vi "PrechargeCurrent.vi"(0 "Storage Voltage In (SP)":sgl format="%#_13g", 1 "Reinitialize":bool=TRUE, 2 "GainP":dbl=0.008 format="%#_13g", 3 "GainI":dbl=0.1 format="%#_13g", 5 "Drive Voltage In (PV)":sgl format="%#_13g", 7 "Setpoint High":dbl=100.0, 9 "Setpoint Low":dbl, 11 "Error In":errorcluster, 12 "Output High":dbl=3.0, 13 "Output Low":dbl) -> (4 "Precharge Current Out":sgl, 15 "Error Out":errorcluster)   [LabVIEW 2014]
uses:
  <vilib>/functionblocks/Control/PID/PID.vi
  <vilib>/functionblocks/FB Core/FB Core.xnode
  <vilib>/functionblocks/NI_FunctionBlock Libraries.lvlib
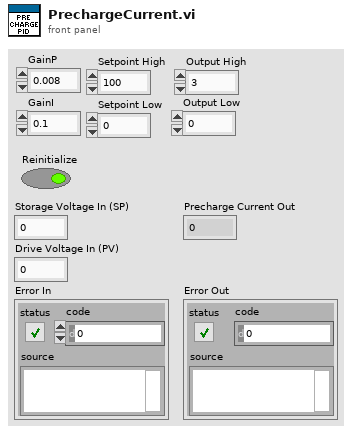
[diagram p1: front panel]
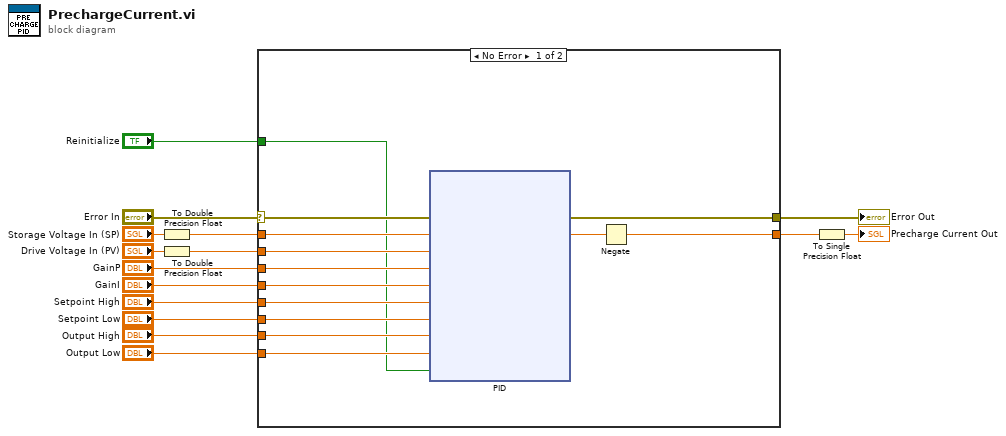
[diagram p0: block diagram]
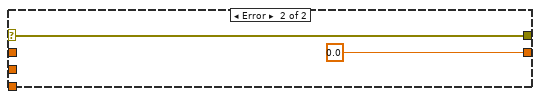
[diagram p2: hidden frame]
diagram:
  n1 = To Double Precision Float(number="Storage Voltage In (SP)") -> (double precision float=w9:dbl)
  n2 = To Double Precision Float(number="Drive Voltage In (PV)") -> (double precision float=w8:dbl)
  n3 = case shown="No Error" "Error In" {
    selector: "Error In" -> [w25 w96]
    tunnel: w9 -> [w28 _]
    tunnel: w8 -> [w27 _]
    tunnel: [w26 w96] -> w13
    tunnel: [w24 0.0 ("output")] -> w12
    tunnel: "Reinitialize" -> [w16 _]
    tunnel: "GainP" -> [w23 _]
    tunnel: "GainI" -> [w22 _]
    tunnel: "Setpoint High" -> [w21 _]
    tunnel: "Setpoint Low" -> [w20 _]
    tunnel: "Output High" -> [w19 _]
    tunnel: "Output Low" -> [w18 _]
    frame No Error {
      n4 = xnode "PID"("error in"=w25, "setpoint"=w28, "process variable"=w27, "proportional gain (Kc)"=w23, "integral time (Ti, min)"=w22, "setpoint high"=w21, "setpoint low"=w20, "output high"=w19, "output low"=w18, "reinitialize? (F)"=w16) -> ("error out"=w26:errorcluster, "output"=w17:dbl)
      n5 = Negate(x=w17) -> (-x=w24:dbl)
    }
    frame Error {
    }
  }
  "Error Out" <- w13
  n6 = To Single Precision Float(number=w12) -> (single precision float=→"Precharge Current Out":sgl)
